vi "ROI preparation.vi"(8 "error in":errorcluster, 9 "ROI":T2, 10 "Width (px)":i32, 11 "Refnum in":T1) -> (0 "error out":errorcluster, 1 "ROI Empty?":bool, 2 "Image Pixels (U8)":u8[][](array[numeric]), 3 "Global Rectangle[0]\nX":i32, 4 "Corrected ROI":u8[][](array[numeric]), 5 "Global Rectangle[1]\nY":i32, 6 "Rect width \n(px)":i32, 7 "Rect height \n(px)":i32)   [LabVIEW 2016]
uses:
  <vilib>/vision/Image Controls.llb/IMAQ Image.ctl
  <vilib>/vision/NI_Vision_Development_Module.lvlib
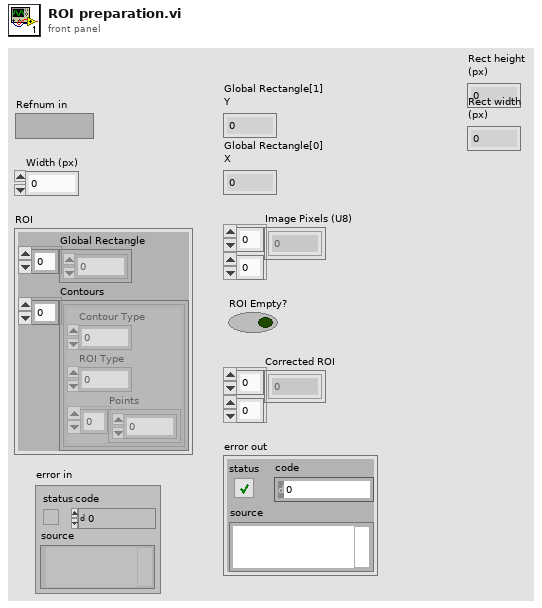
[diagram p1: front panel]
types:
  T1 = typedef "IMAQ Image.ctl" = refnum<image>
  T2 = cluster{"Global Rectangle":i32[], "Contours":cluster{"Contour Type":u32, "ROI Type":u32, "Points":i32[]}[]}
  T3 = typedef "Image Type" = u32
  T4 = cluster{"Global Rectangle[0]":i32, "Global Rectangle[1]":i32}
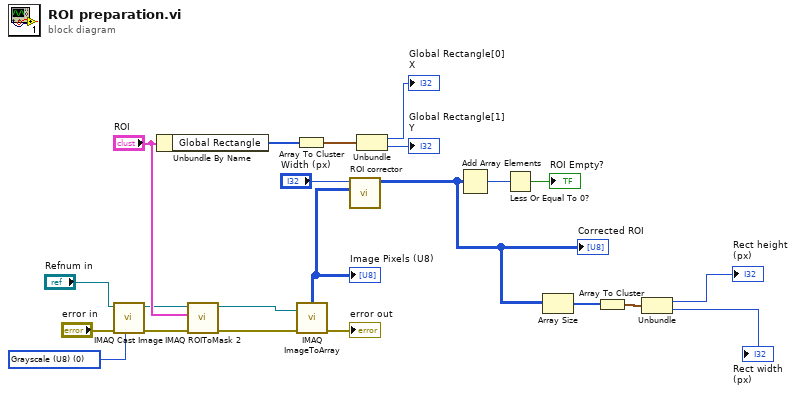
[diagram p0: block diagram]
diagram:
  w10 = T3 0 items=["Grayscale (U8)", "Grayscale (I16)", "Grayscale (SGL)", "Complex (CSG)", "RGB (U32)", "HSL (U32)", "RGB (U64)", "Grayscale (U16)"] ("Image Type")
  n1 = call "IMAQ Cast Image"("Image Type"=w10, "error in (no error)"="error in", "Image Src"="Refnum in") -> ("error out"=w13:errorcluster, "Image Dst Out"=w9:T1)  [unwired: 7 in]
  n2 = Unbundle By Name("ROI") -> ("Global Rectangle"=w18:i32[])
  n3 = call "IMAQ ROIToMask 2"("error in (no error)"=w13, "ROI Descriptor"="ROI", "Image"=w9) -> ("error out"=w12:errorcluster, "Image Out"=w7:T1)  [unwired: 6 in, 1 out]
  n4 = Array To Cluster(array=w18) -> (cluster=w11:T4)
  n5 = call "IMAQ ImageToArray"("error in (no error)"=w12, "Image"=w7) -> ("error out"=→"error out":errorcluster, "Image Pixels (U8)"=w19:u8[][])  [unwired: 2 in, 3 out]
  "Image Pixels (U8)" <- w19
  n6 = call "ROI corrector.vi"("ROI"=w19, "Spot diameter"="Width (px)") -> ("Corrected ROI"=w3:u8[][])  [unwired: 9 in]
  "Corrected ROI" <- w3
  n7 = Unbundle(w11) -> ("Global Rectangle[0]"=→"Global Rectangle[0]\nX":i32, "Global Rectangle[1]"=→"Global Rectangle[1]\nY":i32)
  n8 = Add Array Elements(numeric array=w3) -> (sum=w16:u8)
  n9 = Less Or Equal To 0?(x=w16) -> (x <= 0?=→"ROI Empty?":bool)
  n10 = Array Size(array=w3) -> (size(s)=w5:i32[])
  n11 = Array To Cluster(array=w5) -> (cluster=w4:cluster{"[0]":i32, "[1]":i32})
  n12 = Unbundle(w4) -> ("[0]"=→"Rect height \n(px)":i32, "[1]"=→"Rect width \n(px)":i32)
